vi "Eliminated.vi"(6 "Column":i32, 8 "Row":i32, 9 "Killer":i32, 10 "Team":i32, 11 "Picture In":refnum<class "Picture.lvclass">) -> (3 "Picture Out":refnum<class "Picture.lvclass">)   [LabVIEW 2020, in "Picture.lvclass"]
uses:
  Picture.lvclass
  Picture.lvclass/Picture.ctl
  Squares/Common/Location Data.ctl
  Square/Square.lvclass
  Squares/Common/Common.lvlib
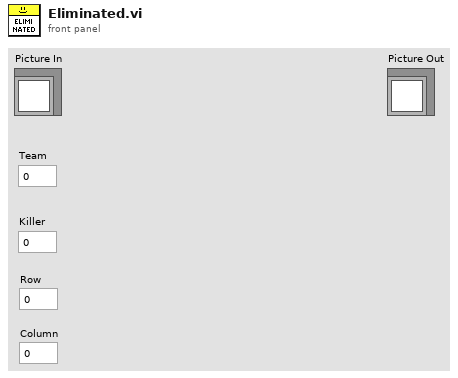
[diagram p1: front panel]
types:
  T1 = typedef "Common.lvlib/Map DVR.ctl" = refnum<data-value>
  T2 = typedef "Common.lvlib/Location Data.ctl" = cluster{"Location State":enum16{"Empty", "Enemy", "Attacked", "Occupied"}, "Round Updated":i32}
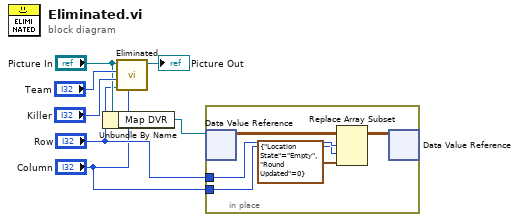
[diagram p0: block diagram]
diagram:
  n1 = Unbundle By Name("Picture In") -> ("Map DVR"=w3:T1)
  n2 = call-parent "Eliminated.vi"("Column"="Column", "Row"="Row", "Killer Index"="Killer", "Team Index"="Team", "Square in"="Picture In") -> ("Square out"=→"Picture Out":refnum<class "Picture.lvclass">)  [unwired: 6 in]
  n3 = in-place {
    in-place-border: "Row" -> [w10]
    in-place-border: "Column" -> [w9]
    n4 = in-place-dvr #1(w3) -> (w12:T2[][])  [unwired: 1 out]
    n5 = Replace Array Subset(array=w12, new element=T2 {"Location State"=enum."Empty", "Round Updated"=0} ("new element/subarray"), index (row)=w10, index (col)=w9) -> (w11:T2[][])
    n6 = in-place-dvr #1(w11) -> ()  [unwired: 2 out]
  }
